vi "Ramp PSU to Magnet.vi"(8 "error in (no error)":errorcluster, 11 "Instrument.Oxford1820 in":refnum<class "Instrument.OxfordVRM.lvclass">) -> (0 "error out":errorcluster, 3 "Instrument.Oxford1820 out":refnum<class "Instrument.OxfordVRM.lvclass">)   [LabVIEW 2016, in "Instrument.OxfordVRM.lvclass"]
uses:
  Instrument.OxfordVRM.lvclass
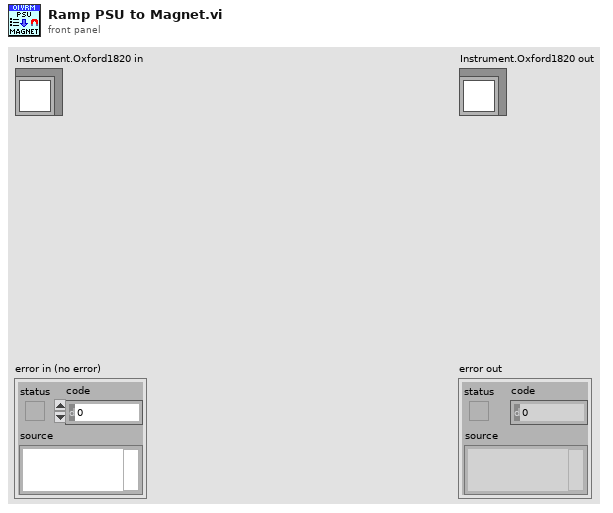
[diagram p1: front panel]
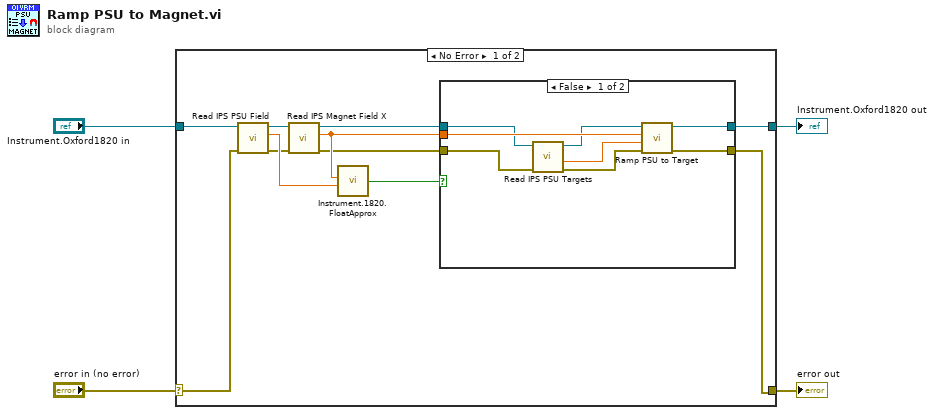
[diagram p0: block diagram]
diagram:
  n1 = case shown="No Error" "error in (no error)" {
    selector: "error in (no error)" -> [w7 w27]
    tunnel: [w14 w27] -> w3
    tunnel: [w15 w26] -> w1
    tunnel: "Instrument.Oxford1820 in" -> [w12 w26]
    frame No Error {
      n2 = call "Read IPS PSU Field.vi"("error in (no error)"=w7, "Instrument.Oxford1820 in"=w12) -> ("error out"=w8:errorcluster, "Power Supply Field (T)"=w11:dbl, "Instrument.Oxford1820 out"=w9:refnum<class "Instrument.OxfordVRM.lvclass">)  [unwired: 7 in]
      n3 = call "Read IPS Magnet Field X.vi"("error in (no error)"=w8, "Instrument.OxfordVRM in"=w9) -> ("error out"=w5:errorcluster, "Magnet Field (T)"=w10:dbl, "Instrument.Oxford1820 out"=w6:refnum<class "Instrument.OxfordVRM.lvclass">)  [unwired: 7 in]
      n4 = call "Instrument.1820.FloatApprox.vi"("y"=w11, "x"=w10) -> ("x ~ y?"=w13:bool)  [unwired: 4 in]
      n5 = case shown="False" w13 {
        tunnel: [w22 w25] -> w15
        tunnel: [w21 w24] -> w14
        tunnel: w6 -> [w19 w25]
        tunnel: w5 -> [w17 w24]
        tunnel: w10 -> [w23 _]
        frame False {
          n6 = call "Read IPS PSU Targets.vi"("error in (no error)"=w17, "Instrument.Oxford1820 in"=w19) -> ("error out"=w16:errorcluster, "Target Field Rate (T/min)"=w20:dbl, "Instrument.Oxford1820 out"=w18:refnum<class "Instrument.OxfordVRM.lvclass">)  [unwired: 6 in, 1 out]
          n7 = call "Ramp PSU to Target.vi"("error in (no error)"=w16, "Target Rate (T/min)"=w20, "Target Field (T)"=w23, "Instrument.Oxford1820 in"=w18) -> ("error out"=w21:errorcluster, "Instrument.Oxford1820 out"=w22:refnum<class "Instrument.OxfordVRM.lvclass">)  [unwired: 6 in]
        }
        frame True {
          # "If PSU == Magnet, do nothing"
        }
      }
    }
    frame Error {
    }
  }
  "error out" <- w3
  "Instrument.Oxford1820 out" <- w1
